vi "mono_gps.vi"(5 "Sensor Connections":T1(array[cluster])) -> (0 "error out":errorcluster, 1 "gps_sample":T2, 2 "tcp_out":refnum<k5>)   [LabVIEW 2018]
panel:
  in  "vertical_acceleration":i32
  in  "horizontal_acceleration":u16
  in  "ego_speed":u16
  in  "ego_yaw":sgl
  in  "forward_z":sgl
  in  "forward_y":sgl
  in  "forward_x":sgl
  in  "location_z":sgl
  in  "location_y":sgl
  in  "location_x":sgl
  in  "elevation":dbl format="%#_13g"
  in  "longitude":dbl format="%#_13g"
  in  "latitude":dbl format="%#_13g"
  in  "payload_length":u8
  in  "sensor_id":u16
  in  "MSG_POS_LLH":u16
  in  "preamble":u8
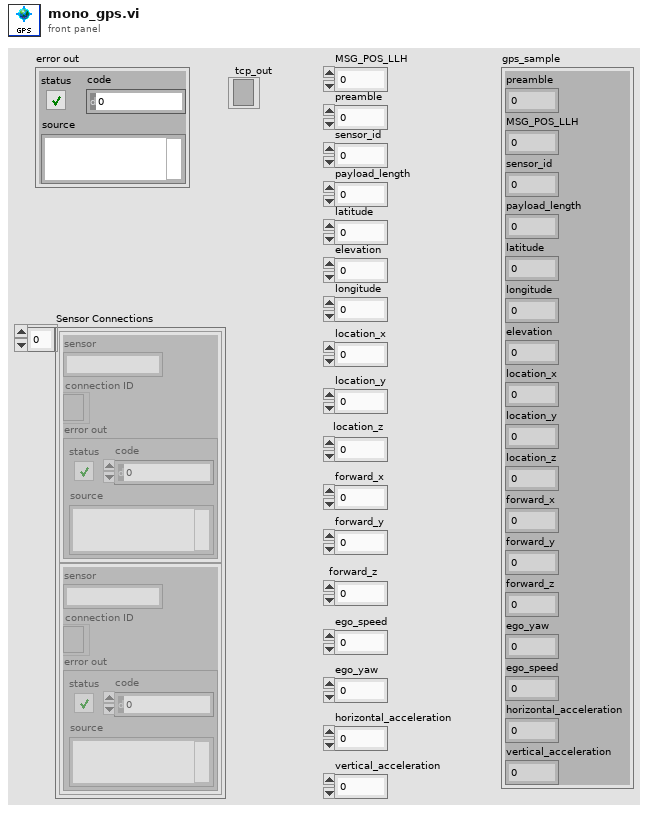
[diagram p1: front panel]
types:
  T1 = cluster{"sensor":string, "connection ID":refnum<k5>, "error out":errorcluster}[]
  T2 = cluster{"preamble":u8, "MSG_POS_LLH":u16, "sensor_id":u16, "payload_length":u8, "latitude":dbl, "longitude":dbl, "elevation":dbl, "location_x":sgl, "location_y":sgl, "location_z":sgl, "forward_x":sgl, "forward_y":sgl, "forward_z":sgl, "ego_yaw":i32, "ego_speed":i32, "horizontal_acceleration":i32, "vertical_acceleration":i32}
  T3 = cluster{"sensor":string, "connection ID":refnum<k5>, "error out":errorcluster}
  T4 = cluster{cluster{"length":u32, "time_stamp":u32, "game_time":sgl}, "data out":string}
  T5 = cluster{"preamble":u8, "MSG_POS_LLH":u16, "sensor_id":u16, "payload_length":u8, "latitude":dbl, "longitude":dbl, "elevation":dbl, "location_x":sgl, "location_y":sgl, "location_z":sgl, "forward_x":sgl, "forward_y":sgl, "forward_z":sgl, "ego_yaw":sgl, "ego_speed":u16, "horizontal_acceleration":u16, "vertical_acceleration":i32}
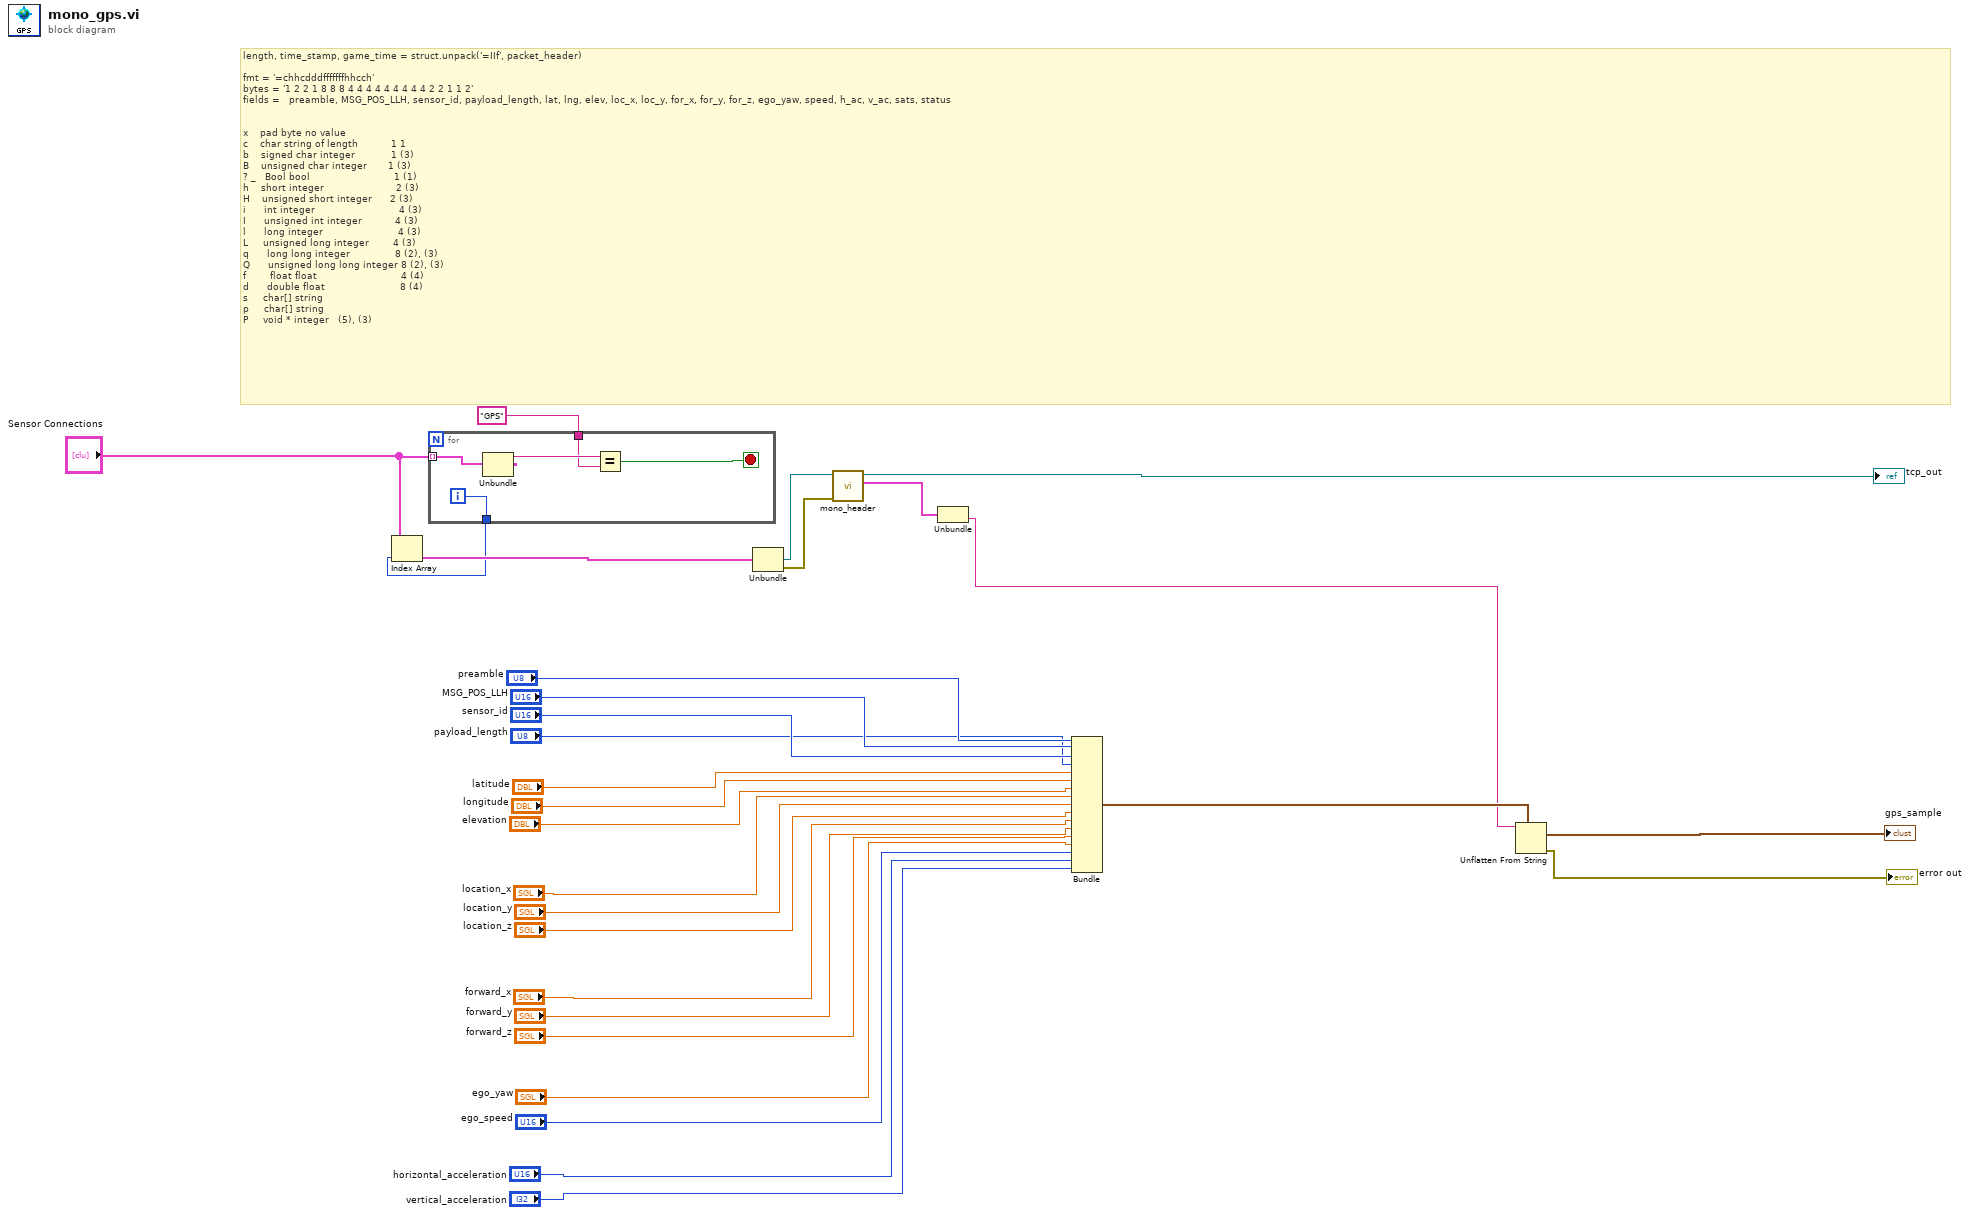
[diagram p0: block diagram]
diagram:
  # "length, time_stamp, game_time = struct.unpack('=IIf', packet_header)\n\nfmt = '=chhcdddfffffffhhcch'\nbytes = '1 2 2 1 8 8 8 4 4 4 4 4 4 4 4 4 2 2 1 1 2'\nfields =   preamble, MSG_POS_LLH, sensor_id, payload_length, lat, lng, elev, loc_x, loc_y, for_x, for_y, for_z, ego_yaw, speed, h_ac, v_ac, sats, status\n\n\nx\t   pad byte\tno value\t \t \nc\t   char\tstring of length           1\t1\t \nb\t   signed char\tinteger\t           1\t(3)\nB\t   unsigned char\tinteger\t      1\t(3)\n?\t_   Bool\tbool\t                           1\t(1)\nh\t   short\tinteger\t                       2\t(3)\nH\t   unsigned short\tinteger\t     2\t(3)\ni\t     int\tinteger\t                           4\t(3)\nI\t     unsigned int\tinteger\t          4\t(3)\nl     \tlong\tinteger\t                        4\t(3)\nL\t    unsigned long\tinteger\t       4\t(3)\nq     \tlong long\tinteger\t              8\t(2), (3)\nQ\t     unsigned long long\tinteger\t8\t(2), (3)\nf       \tfloat\tfloat\t                           4\t(4)\nd     \tdouble\tfloat\t                        8\t(4)\ns\t    char[]\tstring\t \t \np\t    char[]\tstring\t \t \nP\t    void *\tinteger\t \t(5), (3)"
  n1 = for {
    tunnel: "Sensor Connections" -> [w34] mode=indexing
    tunnel: "GPS" -> [w32]
    tunnel: [w30] -> w5
    i -> [w30]
    stop <- w31 stop-if-true
    n2 = Unbundle(w34) -> ("sensor"=w33:string)  [unwired: 2 out]
    n3 = Equal?(x=w33, y=w32) -> (x = y?=w31:bool)
  }
  n4 = Index Array(array="Sensor Connections", index=w5) -> (element=w9:T3)
  n5 = Unbundle(w9) -> ("connection ID"=w7:refnum<k5>, "error out"=w6:errorcluster)  [unwired: 1 out]
  n6 = call "mono_header.vi"("error in"=w6, "connection ID"=w7) -> ("sensor_sample"=w10:T4, "connection ID out"=→"tcp_out":refnum<k5>)  [unwired: 7 in, 1 out]
  n7 = Unbundle(w10) -> ("data out"=w1:string)  [unwired: 1 out]
  n8 = Bundle("preamble"="preamble", "MSG_POS_LLH"="MSG_POS_LLH", "sensor_id"="sensor_id", "payload_length"="payload_length", "latitude"="latitude", "longitude"="longitude", "elevation"="elevation", "location_x"="location_x", "location_y"="location_y", "location_z"="location_z", "forward_x"="forward_x", "forward_y"="forward_y", "forward_z"="forward_z", "ego_yaw"="ego_yaw", "ego_speed"="ego_speed", "horizontal_acceleration"="horizontal_acceleration", "vertical_acceleration"="vertical_acceleration") -> (w29:T5)  [unwired: 1 in]
  n9 = Unflatten From String(type=w29, binary string=w1) -> (value=→"gps_sample":T5, error out=→"error out":errorcluster)  [unwired: 3 in, 1 out]
